vi "Write Buffer 0D I32.vi"(8 "error in (no error)":errorcluster, 9 "offset (0)":u64 format="%d bytes", 10 "src value in":i32, 11 "Buffer in":refnum<class "Buffer.lvclass">) -> (0 "error out":errorcluster, 1 "offset out":u64 format="%d bytes", 2 "src value out":i32, 3 "Buffer out":refnum<class "Buffer.lvclass">)   [LabVIEW 2017, in "DSF Core.lvlib" / "Buffer.lvclass"]
doc: "Writes <b>src value</b> into <b>Buffer</b> at the specified <b>offset</b>."
uses:
  Buffer.lvclass
  C:/Git/DSF/LabVIEW-Memory/Source/Classes/Pointer/Pointer.lvclass
  LabVIEW-Memory/Source/Classes/Pointer/Write I32.vi
  LabVIEW-Memory/Source/Classes/Pointer/Pointer.lvclass
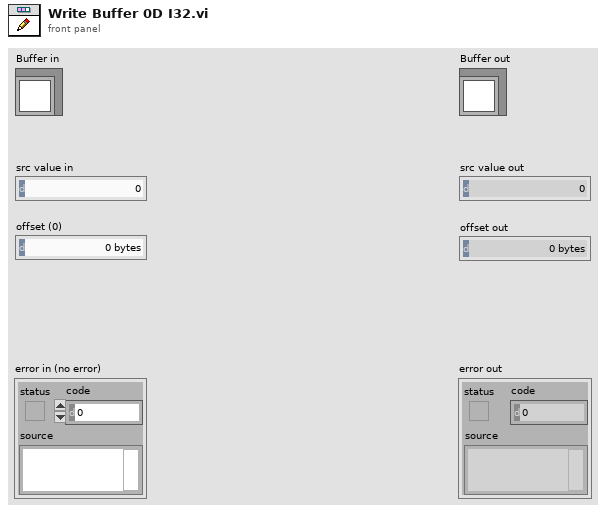
[diagram p1: front panel]
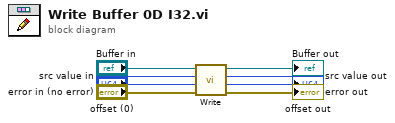
[diagram p0: block diagram]
diagram:
  n1 = call-poly "Write.vi"("error in (no error)"="error in (no error)", "offset (0)"="offset (0)", "value"="src value in", "Pointer in"="Buffer in") -> ("error out"=→"error out":errorcluster, "offset + size"=→"offset out":u64, "value"=→"src value out":i32, "Pointer out"=→"Buffer out":refnum<class "Buffer.lvclass">)  [unwired: 4 in]
